vi "Shooter Mk.II.vi"(2 "Motor":bool, 3 "Fire":bool) -> (0 "Shooter On":bool, 1 "Extend Shooter":bool)   [LabVIEW 2012]
panel:
  in  "Enum":T1(ring)=enum."Shoot"
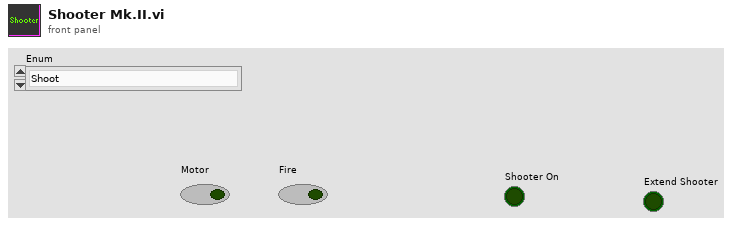
[diagram p1: front panel]
types:
  T1 = enum16{"Start Motor", "Wait 1", "Shoot", "Wait 2", "Retract", "Wait 3"}
  T2 = enum16{"Start Motor", "Wait 1", "Shoot", "Wait 2", "Retract"}
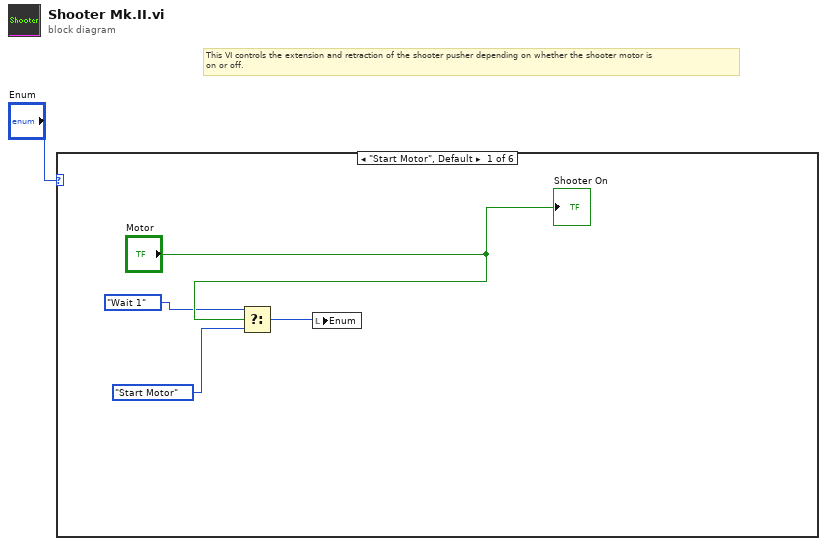
[diagram p0: block diagram]
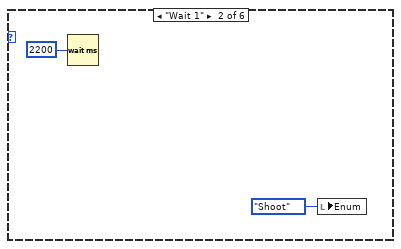
[diagram p2: hidden frame]
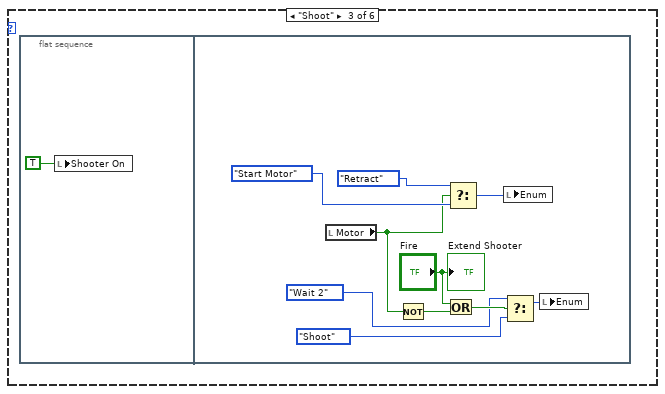
[diagram p3: hidden frame]
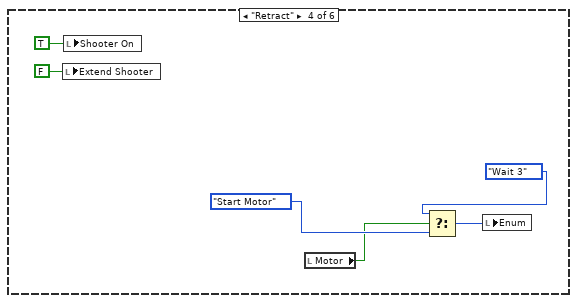
[diagram p4: hidden frame]
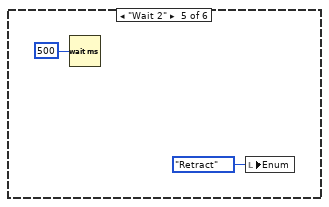
[diagram p5: hidden frame]
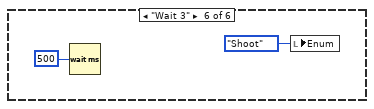
[diagram p6: hidden frame]
diagram:
  # "This VI controls the extension and retraction of the shooter pusher depending on whether the shooter motor is\non or off."
  n1 = case shown="\"Start Motor\", Default" "Enum" {
    frame "Start Motor", Default {
      n2 = Select(t=T2."Wait 1" ("Enum"), s="Motor", f=T2."Start Motor") -> (s? t:f=w4:T2)
      n3 = local write "Enum"(w4) -> ()
      "Shooter On" <- "Motor"
    }
    frame "Wait 1" {
      n4 = Wait (ms)(milliseconds to wait=u32 2200) -> ()  [unwired: 1 out]
      n5 = local write "Enum"(T2."Shoot" ("Enum")) -> ()
    }
    frame "Shoot" {
      n6 = flat-sequence {
        frame #0 {
          n7 = local write "Shooter On"(TRUE ("Shooter On")) -> ()
        }
        frame #1 {
          n8 = local read "Motor"() -> (w9:bool)
          n9 = Not(x=w9) -> (.not. x?=w17:bool)
          n10 = Or(x="Fire", y=w17) -> (x .or. y?=w15:bool)
          n11 = Select(t=T2."Retract" ("Enum"), s=w9, f=T1."Start Motor" ("Enum")) -> (s? t:f=w11:T1)
          n12 = local write "Enum"(w11) -> ()
          n13 = Select(t=T2."Wait 2" ("Enum"), s=w15, f=T2."Shoot" ("Enum")) -> (s? t:f=w14:T2)
          n14 = local write "Enum"(w14) -> ()
          "Extend Shooter" <- "Fire"
        }
      }
    }
    frame "Retract" {
      n15 = local write "Extend Shooter"(FALSE ("Extend Shooter")) -> ()
      n16 = local write "Shooter On"(TRUE ("Shooter On")) -> ()
      n17 = local read "Motor"() -> (w20:bool)
      n18 = Select(t=T1."Wait 3" ("Enum"), s=w20, f=T1."Start Motor" ("Enum")) -> (s? t:f=w22:T1)
      n19 = local write "Enum"(w22) -> ()
    }
    frame "Wait 2" {
      n20 = Wait (ms)(milliseconds to wait=u32 500) -> ()  [unwired: 1 out]
      n21 = local write "Enum"(T2."Retract" ("Enum")) -> ()
    }
    frame "Wait 3" {
      n22 = Wait (ms)(milliseconds to wait=u32 500) -> ()  [unwired: 1 out]
      n23 = local write "Enum"(T1."Shoot" ("Enum")) -> ()
    }
  }
